vi "test Add Script Deploy.vi"(8 "error in":errorcluster, 11 "TestCase in":refnum<class "Examples.lvclass">) -> (0 "error out":errorcluster, 3 "TestCase out":refnum<class "Examples.lvclass">)   [LabVIEW 2020, in "Examples.lvclass"]
uses:
  Examples.lvclass
  C:/Git/niveristand-custom-device-testing-tools/VeriStandTestCase/VeriStandTestCase.lvclass
  Examples.lvclass/Examples.ctl
  7f6914e5-79d7-41a5-a6cd-be6651e4326d.vi
  <vilib>/addons/_JKI Toolkits/VI Tester/TestCase.llb/TestCase.lvclass
  C:/Program Files (x86)/National Instruments/LabVIEW 2020/vi.lib/addons/_JKI Toolkits/VI Tester/TestCase.llb/TestCase.lvclass
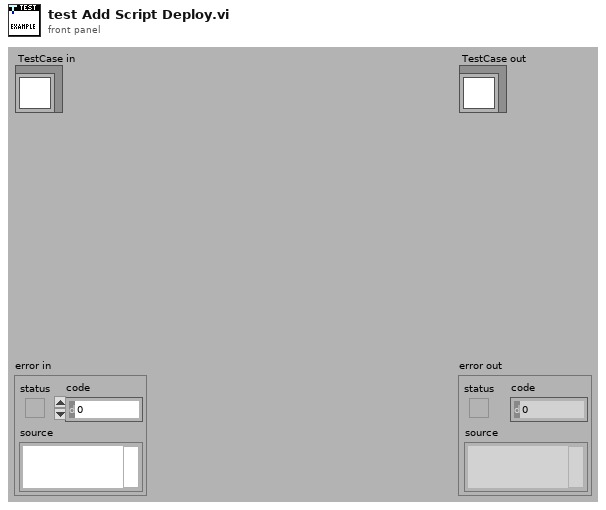
[diagram p1: front panel]
types:
  T1 = typedef "NI_VS Workspace ExecutionAPI.lvlib/WorkspaceAPI.ctl" = refnum<k24>
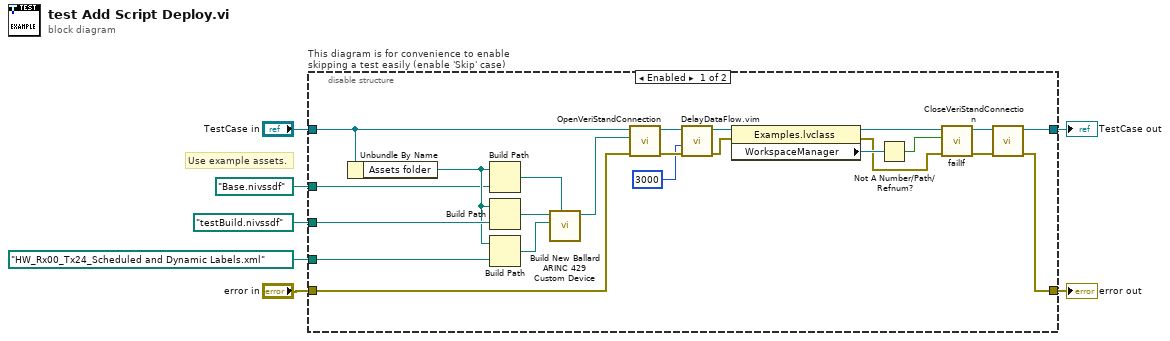
[diagram p0: block diagram]
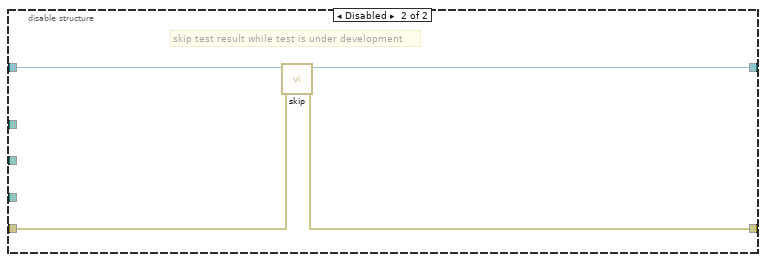
[diagram p2: hidden frame]
diagram:
  # "Use example assets."
  n1 = disable-structure "This diagram is for convenience to enable skipping a test easily (enable 'Skip' case)" shown="Enabled" {
    disable-tunnel: "TestCase in" -> [w17 w33]
    disable-tunnel: [w18 w31] -> w4
    disable-tunnel: [w19 w32] -> w6
    disable-tunnel: "error in" -> [w8 w30]
    disable-tunnel: path "HW_Rx00_Tx24_Scheduled and Dynamic Labels.xml" ("name or relative path") -> [w16 _]
    disable-tunnel: path "testBuild.nivssdf" ("name or relative path") -> [w15 _]
    disable-tunnel: path "Base.nivssdf" ("name or relative path") -> [w11 _]
    frame Enabled {
      n2 = Unbundle By Name(w17) -> ("Assets folder"=w12:path)
      n3 = Build Path(base path=w12, name or relative path=w11) -> (appended path=w10:path)
      n4 = Build Path(base path=w12, name or relative path=w15) -> (appended path=w14:path)
      n5 = Build Path(base path=w12, name or relative path=w16) -> (appended path=w13:path)
      n6 = call "Build New Ballard ARINC 429 Custom Device.vi"("Base System Definition File"=w10, "Hardware Configuration File"=w13, "Output System Definition File"=w14) -> ("Ballard ARINC 429 System Definition"=w9:path)  [unwired: 8 in]
      n7 = call-dynamic "OpenVeriStandConnection.vi"("error in (no error)"=w8, "System Definition File"=w9, "VeriStand Test Case in"=w17) -> ("error out"=w22:errorcluster, "VeriStand Test Case out"=w21:refnum<class "Examples.lvclass">)  [unwired: 6 in, 1 out]
      n8 = call "DelayDataFlow.vim"("value in"=w22, "milliseconds to wait"=u32 3000) -> ("value out"=w29:errorcluster)  [unwired: 2 in, 1 out]
      n9 = property class="Examples.lvclass"(reference=w21, error in=w29) -> (reference out=w28:refnum<class "Examples.lvclass">, error out=w23:errorcluster, "WorkspaceManager"=w25:T1)
      n10 = Not A Number/Path/Refnum?(number/path/refnum=w25) -> (NaN/Path/Refnum?=w24:bool)
      n11 = call-dynamic "failIf.vi"("error in (no error)"=w23, "fail"=w24, "TestCase in"=w28) -> ("error out"=w26:errorcluster, "TestCase out"=w27:refnum<class "Examples.lvclass">)  [unwired: 7 in]
      n12 = call-dynamic "CloseVeriStandConnection.vi"("error in (no error)"=w26, "VeriStand Test Case in"=w27) -> ("error out"=w19:errorcluster, "VeriStand Test Case out"=w18:refnum<class "Examples.lvclass">)  [unwired: 8 in]
    }
    frame Disabled {
      # "skip test result while test is under development"
      n13 = call <vilib>:"skip.vi"("error in (no error)"=w30, "TestCase in"=w33) -> ("error out"=w32:errorcluster, "TestCase out"=w31:refnum<class "Examples.lvclass">)  [unwired: 8 in]
    }
  }
  "error out" <- w6
  "TestCase out" <- w4
